vi "ActorDB-PerformUpdateAllInstruction.vi"(5 "SQL Statement":string, 6 "Cluster In":T1(array[cluster]), 7 "Update All":bool, 8 "error in (no error)":errorcluster, 9 "Column Number":i32, 10 "Table":string, 11 "Database-API in":refnum<class "PartCertDatabase-API.lvclass">) -> (0 "error out":errorcluster, 2 "New SQL Statement":string, 3 "Database-API out":refnum<class "PartCertDatabase-API.lvclass">)   [LabVIEW 2013, in "PartCertDatabase-Actor.lvclass"]
uses:
  PartCertDatabase-Actor.lvclass
  Reuse Library/Database API/PartCertDatabase-API.lvclass
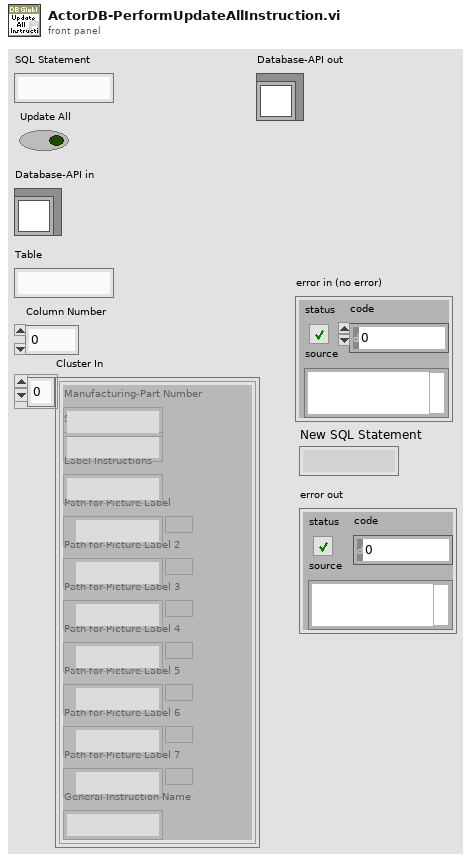
[diagram p1: front panel]
types:
  T1 = cluster{"Manufacturing-Part Number":string, "Step Number":string, "Label Instructions":string, "Path for Picture Label":path, "Path for Picture Label 2":path, "Path for Picture Label 3":path, "Path for Picture Label 4":path, "Path for Picture Label 5":path, "Path for Picture Label 6":path, "Path for Picture Label 7":path, "General Instruction Name":string}[]
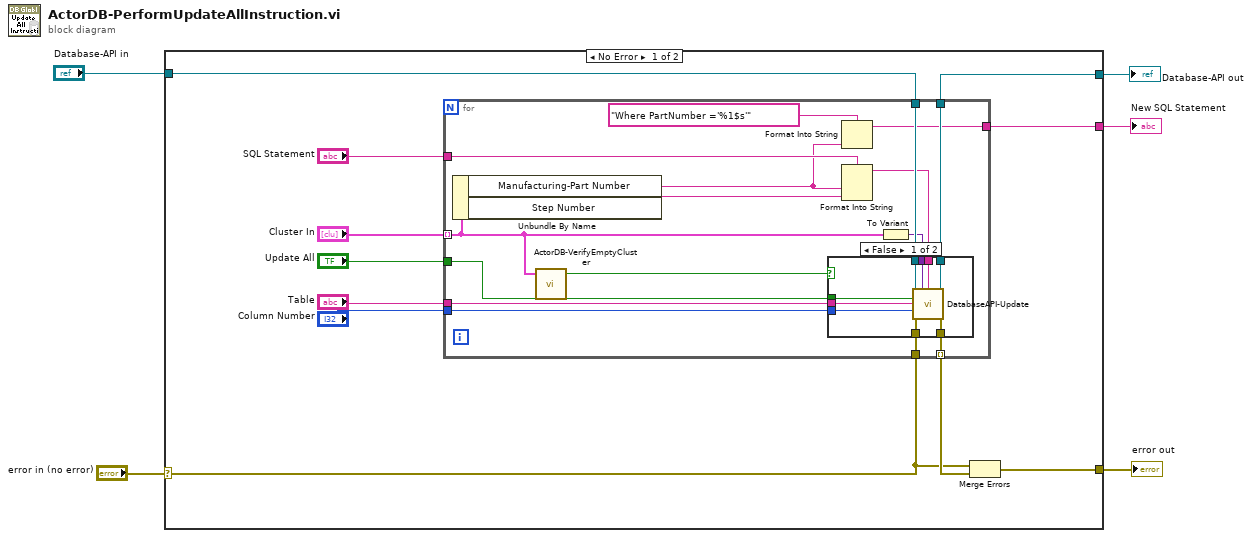
[diagram p0: block diagram]
diagram:
  n1 = case shown="No Error" "error in (no error)" {
    selector: "error in (no error)" -> [w6 w45]
    tunnel: [w13 w44] -> w5
    tunnel: "Database-API in" -> [w10 w44]
    tunnel: [w9 _] -> w3
    tunnel: [w7 w45] -> w2
    frame No Error {
      n2 = for {
        tunnel: w10 -> [w32]
        tunnel: "Update All" -> [w31]
        tunnel: "SQL Statement" -> [w20]
        tunnel: [w30] -> w13
        tunnel: "Table" -> [w29]
        tunnel: [w28] -> w8 mode=indexing
        tunnel: "Column Number" -> [w27]
        tunnel: w6 -> [w26]
        tunnel: "Cluster In" -> [w23] mode=indexing
        tunnel: [w18] -> w9
        n3 = Unbundle By Name(w23) -> ("Manufacturing-Part Number"=w17:string, "Step Number"=w21:string)
        n4 = call "ActorDB-VerifyEmptyCluster.vi"("Cluster In"=w23) -> ("Don't Run Update"=w22:bool)  [unwired: 8 in]
        n5 = Format Into String(format string="Where PartNumber ='%1$s'", w17) -> (resulting string=w18:string)  [unwired: 2 in, 1 out]
        n6 = Format Into String(format string=w20, w17, w21) -> (resulting string=w24:string)  [unwired: 2 in, 1 out]
        n7 = To Variant(anything=w23) -> (Variant=w25:variant)
        n8 = case shown="False" w22 {
          tunnel: w32 -> [w41 w43]
          tunnel: w31 -> [w40 _]
          tunnel: [w39 w43] -> w30
          tunnel: w29 -> [w38 _]
          tunnel: [w37 w42] -> w28
          tunnel: w27 -> [w36 _]
          tunnel: w26 -> [w35 w42]
          tunnel: w25 -> [w34 _]
          tunnel: w24 -> [w33 _]
          frame False {
            n9 = call "DatabaseAPI-Update.vi"("Database-API in"=w41, "data"=w34, "Where Statement"=w33, "Update All"=w40, "Table"=w38, "Column Number"=w36, "error in (no error)"=w35) -> ("Database-API out"=w39:refnum<class "PartCertDatabase-API.lvclass">, "error out"=w37:errorcluster)  [unwired: 7 in]
          }
          frame True {
          }
        }
      }
      n10 = Merge Errors(w6, w8) -> (w7:errorcluster)
    }
    frame Error {
    }
  }
  "Database-API out" <- w5
  "New SQL Statement" <- w3
  "error out" <- w2
